vi "read_curve_properties.vi"(10 "data_type":enum16{"Nanopuller", "Agilent", "Bioscope"}(ring), 11 "current_curve":path) -> (0 "deflection_sensitivity":dbl, 1 "force_constant":dbl, 2 "um":bool, 3 "nN":bool)   [LabVIEW 2015]
uses:
  <vilib>/Utility/file.llb/Read Delimited Spreadsheet (string).vi
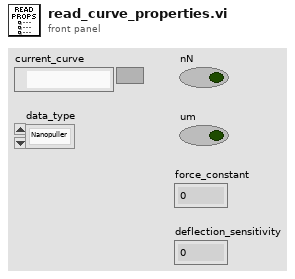
[diagram p1: front panel]
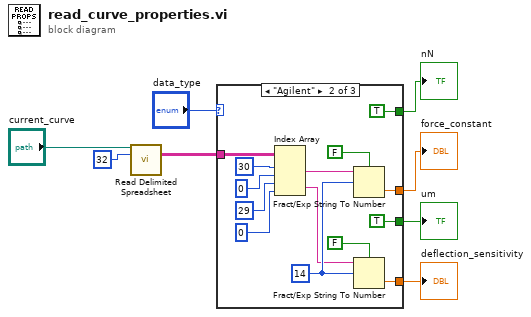
[diagram p0: block diagram]
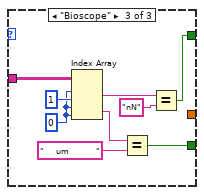
[diagram p3: hidden frame]
diagram:
  n1 = call-poly <vilib>:"Read Delimited Spreadsheet.vi"("file path (dialog if empty)"="current_curve", "number of rows (all:-1)"=32) -> ("all rows"=w3:string[][])  [unwired: 8 in, 5 out]
  n2 = case shown="\"Agilent\"" "data_type" {
    tunnel: [_ TRUE w28] -> w1
    tunnel: [_ TRUE w24] -> w2
    tunnel: w3 -> [_ w16 w23]
    tunnel: [_ w10 _] -> w7
    tunnel: [_ w9 _] -> w8
    frame "Nanopuller", Default {
    }
    frame "Agilent" {
      w12 = 14 ("offset (0)")
      n3 = Index Array(array=w16, index (row) #1=30 ("index (row)"), index (col) #1=0 ("disabled index (col)"), index (row) #2=29 ("index (row)"), index (col) #2=0 ("index (row)")) -> (element #1=w13:string, element #2=w11:string)
      n4 = Fract/Exp String To Number(use system decimal point (T)=FALSE, string=w13, offset=w12) -> (number=w10:dbl)  [unwired: 1 in, 1 out]
      n5 = Fract/Exp String To Number(use system decimal point (T)=FALSE, string=w11, offset=w12) -> (number=w9:dbl)  [unwired: 1 in, 1 out]
    }
    frame "Bioscope" {
      w27 = 0 ("index (row)")
      n6 = Index Array(array=w23, index (row) #1=w27, index (col) #1=1 ("disabled index (col)"), index (row) #2=w27, index (col) #2=w27) -> (element #1=w30:string, element #2=w25:string)
      n7 = Equal?(x=w25, y="    um         ") -> (x = y?=w24:bool)
      n8 = Equal?(x=w30, y="nN") -> (x = y?=w28:bool)
    }
  }
  "deflection_sensitivity" <- w8
  "force_constant" <- w7
  "um" <- w2
  "nN" <- w1
